vi "Init.vi"(8 "error in (no error)":errorcluster, 10 "Slot Name":string, 11 "Data Realm":T1) -> (0 "error out":errorcluster, 3 "GetPersistentData out":refnum<class "GetPersistentData.lvclass">)   [LabVIEW 2022 SP3, in "obs-websocket-lv.lvlib" / "GetPersistentData.lvclass"]
uses:
  GetPersistentData.lvclass
  GetPersistentData.lvclass/GetPersistentData.ctl
  Data Realm.ctl
  obs-websocket-lv.lvlib
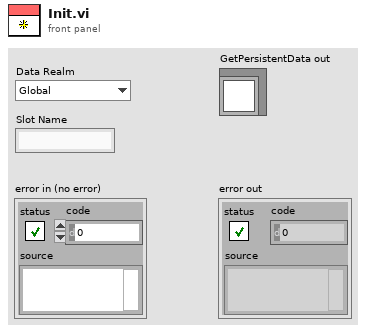
[diagram p1: front panel]
types:
  T1 = typedef "obs-websocket-lv.lvlib/Data Realm.ctl" = enum16{"Global", "Profile"}
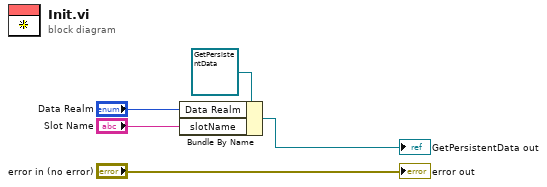
[diagram p0: block diagram]
diagram:
  n1 = Bundle By Name(cluster=refnum<class "GetPersistentData.lvclass"> refnum ("GetPersistentData in"), "Data Realm"="Data Realm", "slotName"="Slot Name") -> (→"GetPersistentData out":refnum<class "GetPersistentData.lvclass">)
  "error out" <- "error in (no error)"
